vi "init.vi"(8 "error in (no error)":errorcluster, 11 "WeatherData.lvclass":refnum<class "WeatherData.lvclass">) -> (0 "error out":errorcluster, 3 "WeatherData.lvclass 2":refnum<class "WeatherData.lvclass">)   [LabVIEW 2020, in "WeatherData.lvclass"]
uses:
  WeatherData.lvclass
  weatherDataCluster.ctl
  Observer/Observer.lvclass
  WeatherData.lvclass/WeatherData.ctl
panel:
  # "Connector Pane"
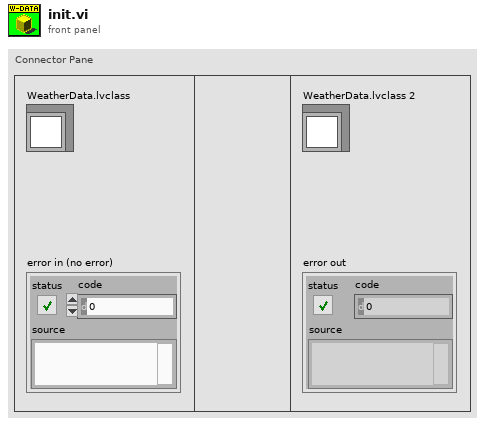
[diagram p1: front panel]
types:
  T1 = typedef "WeatherData.lvclass/weatherDataCluster.ctl" = cluster{"Temperature":dbl, "Humidity":dbl, "Pressure":dbl, "Observers":refnum<class "Observer.lvclass">[]}
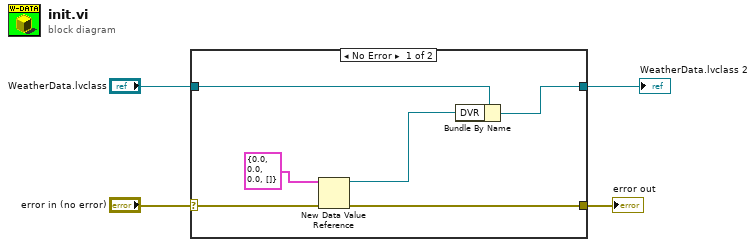
[diagram p0: block diagram]
diagram:
  n1 = case shown="No Error" "error in (no error)" {
    selector: "error in (no error)" -> [w10 w11]
    tunnel: [w5 w11] -> w3
    tunnel: [w6 w12] -> w2
    tunnel: "WeatherData.lvclass" -> [w8 w12]
    frame No Error {
      n2 = New Data Value Reference(data value=T1 {"Temperature"=0.0, "Humidity"=0.0, "Pressure"=0.0, "Observers"=[]} ("Cluster of class private data"), error in=w10) -> (data value reference=w7:refnum<data-value>, error out=w5:errorcluster)
      n3 = Bundle By Name(cluster=w8, "DVR"=w7) -> (w6:refnum<class "WeatherData.lvclass">)
    }
    frame Error {
    }
  }
  "WeatherData.lvclass 2" <- w2
  "error out" <- w3
